vi "Read Results from processing.vi"(8 "error in":errorcluster, 11 "ActiveFrontEndModule runtime in":refnum<class "ActiveFrontEndModule runtime.lvclass">) -> (0 "error out":errorcluster, 2 "Results from processing":T1, 3 "ActiveFrontEndModule runtime out":refnum<class "ActiveFrontEndModule runtime.lvclass">)   [LabVIEW 2017, in "ActiveFrontEndModule runtime.lvclass"]
uses:
  ActiveFrontEndModule runtime.lvclass
  configuration/result data indices.ctl
  ActiveFrontEndModule runtime.lvclass/ActiveFrontEndModule runtime.ctl
  configuration/ActiveFrontEndModule configuration.lvclass
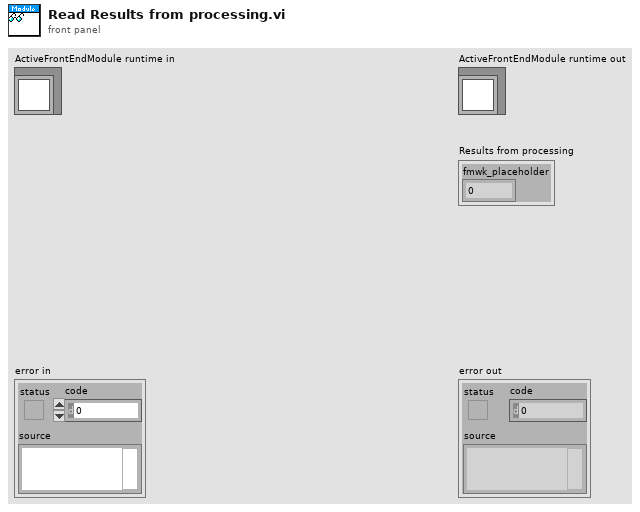
[diagram p1: front panel]
types:
  T1 = typedef "ActiveFrontEndModule configuration.lvclass/result data indices.ctl" = cluster{"fmwk_placeholder":i32}
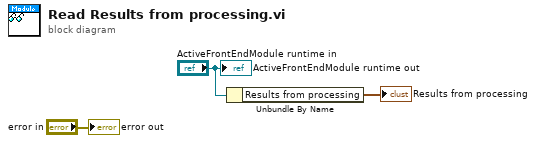
[diagram p0: block diagram]
diagram:
  n1 = Unbundle By Name("ActiveFrontEndModule runtime in") -> ("Results from processing"=→"Results from processing":T1)
  "error out" <- "error in"
  "ActiveFrontEndModule runtime out" <- "ActiveFrontEndModule runtime in"
